vi "Shift by Site.vi"(11 "Location":string) -> (3 "Shift":i32)   [LabVIEW 2017]
panel:
  out "date/time string":string
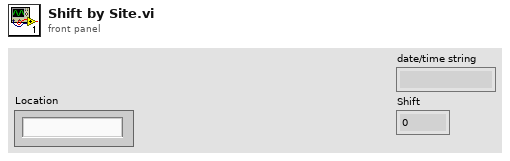
[diagram p1: front panel]
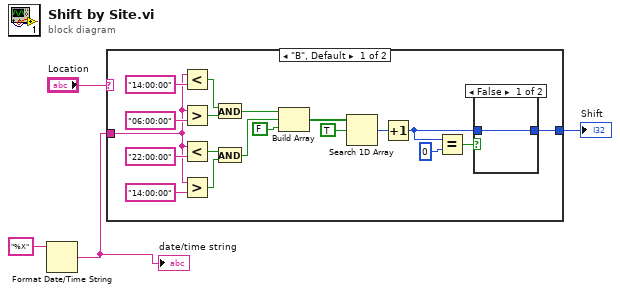
[diagram p0: block diagram]
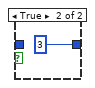
[diagram p2: hidden frame]
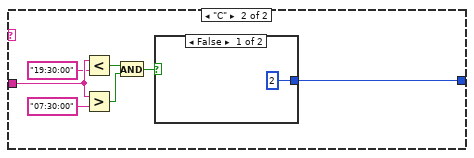
[diagram p3: hidden frame]
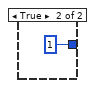
[diagram p4: hidden frame]
diagram:
  n1 = Format Date/Time String(time format string (%c)="%X") -> (date/time string=w1:string)  [unwired: 2 in]
  "date/time string" <- w1
  n2 = case shown="\"B\", Default" "Location" {
    tunnel: w1 -> [w15 w31]
    tunnel: [w6 w26] -> w2
    frame "B", Default {
      n3 = Less?(x=w15, y="14:00:00") -> (x < y?=w20:bool)
      n4 = Greater?(x=w15, y="06:00:00") -> (0:w21:bool)
      n5 = Less?(x=w15, y="22:00:00") -> (x < y?=w16:bool)
      n6 = Greater?(x=w15, y="14:00:00") -> (0:w17:bool)
      n7 = And(x=w20, y=w21) -> (x .and. y?=w14:bool)
      n8 = And(x=w16, y=w17) -> (x .and. y?=w13:bool)
      n9 = Build Array(w14, w13, FALSE ("element")) -> (w12:bool[])
      n10 = Search 1D Array(1D array=w12, element=TRUE) -> (index of element=w10:i32)  [unwired: 1 in]
      n11 = Increment(x=w10) -> (x+1=w5:i32)
      n12 = Equal?(x=w5, y=0) -> (x = y?=w8:bool)
      n13 = case shown="False" w8 {
        tunnel: [w24 3 ("y")] -> w6
        tunnel: w5 -> [w24 _]
        frame False {
        }
        frame True {
        }
      }
    }
    frame "C" {
      n14 = Less?(x=w31, y="19:30:00") -> (x < y?=w29:bool)
      n15 = Greater?(x=w31, y="07:30:00") -> (0:w28:bool)
      n16 = And(x=w29, y=w28) -> (x .and. y?=w27:bool)
      n17 = case shown="False" w27 {
        tunnel: [2 1] -> w26
        frame False {
        }
        frame True {
        }
      }
    }
  }
  "Shift" <- w2
